vi "Write Device Identification.vi"(7 "unit ID":u8, 8 "error in":errorcluster, 10 "objects":T1[](array[typedef]) {"Object ID" format="%x"}, 11 "Modbus slave in":refnum<class "Modbus Slave.lvclass">) -> (0 "error out":errorcluster, 3 "Modbus slave out":refnum<class "Modbus Slave.lvclass">)   [LabVIEW 2013, in "Modbus Library - Advance.lvlib" / "Modbus Slave.lvclass"]
doc: "Writes Modbus object information stored on the device. This can include basic information, like manufacturer, additional standard items, or model-specific extended items. This function may take a large amount of time to execute, as it requires the transfer of a large quantity of binary data. Even on TCP/IP, this function is limited by the maximum defined size of a Modbus protocol data unit. If a slave supports objects, it is required that it stores information for VendorName (0x00), ProductCode (0x01), and MajorMinorRevision (0x02). The standard device data model provided by this library accepts any object request and can store any objects."
uses:
  Modbus Slave.lvclass
  Data Model/Identification Parameters.ctl
  Modbus Slave.lvclass/Modbus Slave.ctl
  Standard Data Model/Standard Data Model.lvclass
  Super Data Model/Super Data Model.lvclass
  Data Model/Device Data Model.lvclass
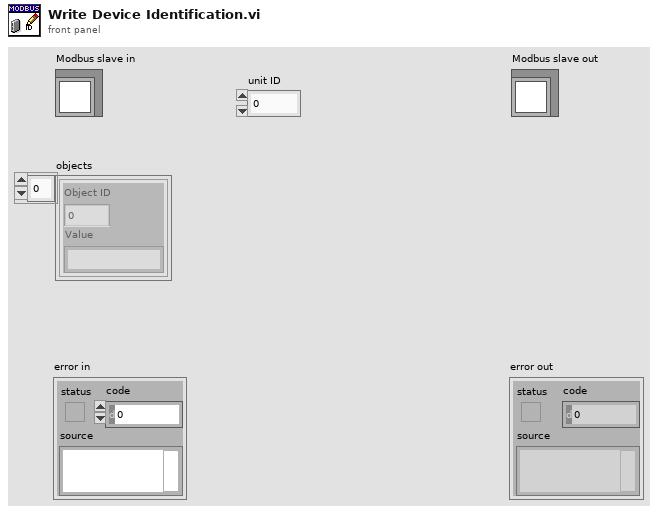
[diagram p1: front panel]
types:
  T1 = typedef "Modbus Library - Advance.lvlib/Device Data Model.lvclass/Identification Parameters.ctl" = cluster{"Object ID":u8, "Value":string}
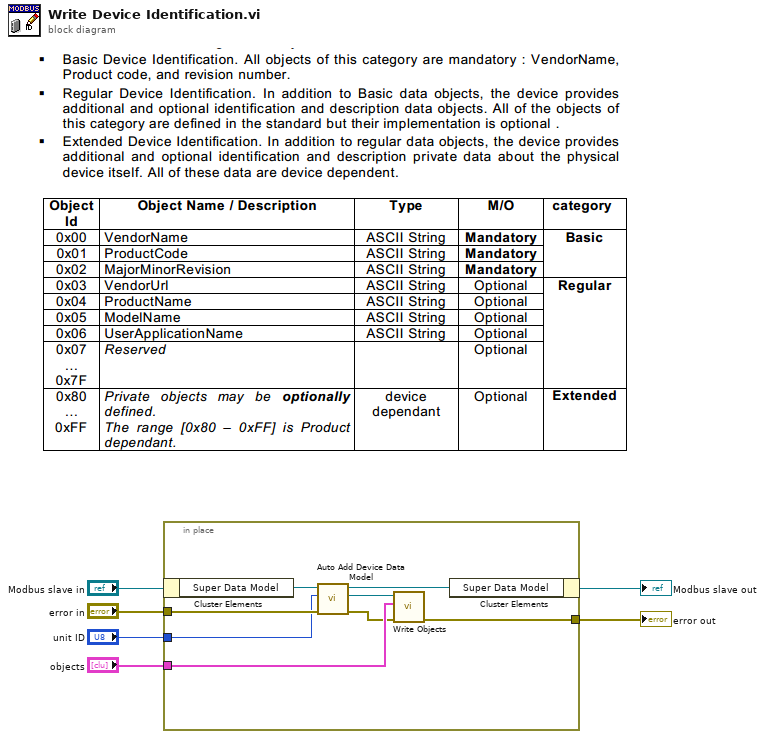
[diagram p0: block diagram]
diagram:
  n1 = in-place {
    in-place-border: [w14] -> w4
    in-place-border: "objects" -> [w13]
    in-place-border: "error in" -> [w11]
    in-place-border: "unit ID" -> [w10]
    n2 = in-place-cluster #1("Modbus slave in") -> ("Super Data Model"=w12:refnum<class "Super Data Model.lvclass">)
    n3 = call "Auto Add Device Data Model.vi"("error in"=w11, "unit ID"=w10, "Super Data Model in"=w12) -> ("error out"=w8:errorcluster, "device data model"=w9:refnum<class "Standard Data Model.lvclass">, "Super Data Model out"=w7:refnum<class "Super Data Model.lvclass">)  [unwired: 6 in]
    n4 = call-dynamic "Write Objects.vi"("error in"=w8, "Objects"=w13, "Standard Data Model in"=w9) -> ("error out"=w14:errorcluster)  [unwired: 7 in, 1 out]
    n5 = in-place-cluster #1("Super Data Model"=w7) -> (→"Modbus slave out":refnum<class "Modbus Slave.lvclass">)
  }
  "error out" <- w4
